vi "Download GitHub Resource.vi"(7 "Output file":path, 8 "error in (no error)":errorcluster, 11 "URL":string) -> (0 "error out":errorcluster)   [LabVIEW 2020]
uses:
  <vilib>/httpClient/LabVIEWHTTPClient.lvlib
  <vilib>/regexp/Match Regular Expression.xnode
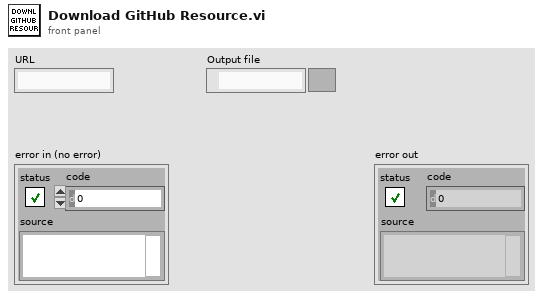
[diagram p1: front panel]
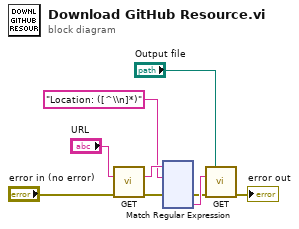
[diagram p0: block diagram]
diagram:
  n1 = call <vilib>:"GET.vi"("url"="URL", "error in (no error)"="error in (no error)") -> ("headers"=w8:string, "error out"=w4:errorcluster)  [unwired: 10 in, 2 out]
  n2 = xnode "Match Regular Expression"("input string"=w8, "regular expression"="Location: ([^\\n]*)", "error in"=w4) -> ("error out"=w3:errorcluster, "submatch 1"=w5:string)  [unwired: 3 in, 4 out]
  n3 = call <vilib>:"GET.vi"("output file"="Output file", "url"=w5, "error in (no error)"=w3) -> ("error out"=→"error out":errorcluster)  [unwired: 9 in, 3 out]
